vi "ROI group-Update All Groups info.vi"(8 "error in (no error)":errorcluster, 11 "Groups setup to add/update":T1[](array[typedef]) {"Group region specifier cluster"."Contours"."Type" items=["No Selection", "Point", "Line", "Rectangle", "Oval", "Polygon", "Freehand Region", "Annulus", "Unused2", "Unused3", "Broken Line", "Freehand Line", "Rotated Rectangle"]}) -> (0 "error out":errorcluster, 3 "Updated \"All groups\" setup":T1[](array[typedef]) {"Group region specifier cluster"."Contours"."Type" items=["No Selection", "Point", "Line", "Rectangle", "Oval", "Polygon", "Freehand Region", "Annulus", "Unused2", "Unused3", "Broken Line", "Freehand Line", "Rotated Rectangle"]})   [LabVIEW 2013]
uses:
  ROI Selection Interface/ROI group info cluster.ctl
  Typedefs/Get-Set-Clear Control.ctl
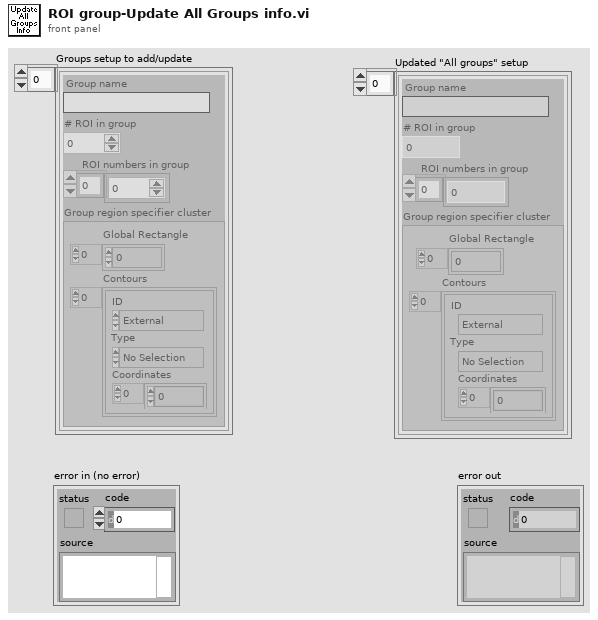
[diagram p1: front panel]
types:
  T1 = typedef "ROI group info cluster.ctl" = cluster{"Group name":string, "# ROI in group":i32, "ROI numbers in group":i32[], "Group region specifier cluster":T2}
  T2 = typedef "ROI Descriptor" = cluster{"Global Rectangle":i32[], "Contours":cluster{"ID":enum32{"External", "Internal"}, "Type":u32, "Coordinates":i32[]}[]}
  T3 = typedef "Get-Set-Clear Control.ctl" = enum16{"Get", "Set", "Clear"}
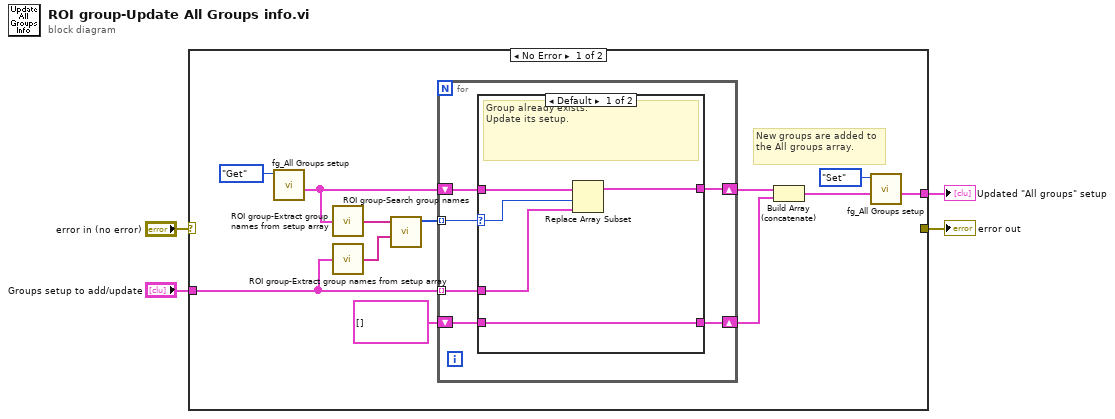
[diagram p0: block diagram]
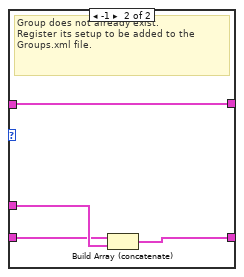
[diagram p2: hidden frame]
diagram:
  n1 = case shown="No Error" "error in (no error)" {
    selector: "error in (no error)" -> [_ w32]
    tunnel: "Groups setup to add/update" -> [w11 _]
    tunnel: [w5 _] -> w3
    tunnel: [_ w32] -> w1
    frame No Error {
      # "New groups are added to the All groups array."
      n2 = call "fg_All Groups setup.vi"("Function"=Get-Set-Clear_Control."Get") -> ("Groups setup out"=w12:T1[])  [unwired: 9 in, 1 out]
      n3 = call "ROI group-Extract group names from setup array.vi"("Groups setup"=w12) -> ("Group Names Array"=w15:string[])
      n4 = call "ROI group-Extract group names from setup array.vi"("Groups setup"=w11) -> ("Group Names Array"=w14:string[])
      n5 = call "ROI group-Search group names.vi"("Group names to search for"=w14, "Group names to search through"=w15) -> ("Indexes (-1 = not found)"=w13:i32[])  [unwired: 9 in]
      n6 = for {
        tunnel: w13 -> [w22] mode=indexing
        tunnel: w11 -> [w20] mode=indexing
        shift-right: [w19] -> w9
        shift-left: w12 -> [w21]
        shift-right: [w18] -> w8
        shift-left: T1[] [] -> [w17]
        n7 = case shown="Default" w22 {
          selector: w22 -> [w26 _]
          tunnel: w21 -> [w27 w31]
          tunnel: w20 -> [w25 w30]
          tunnel: [w24 w31] -> w19
          tunnel: [w23 w29] -> w18
          tunnel: w17 -> [w23 w28]
          frame Default {
            # "Group already exists.\nUpdate its setup."
            n8 = Replace Array Subset(array=w27, new element=w25, index=w26) -> (w24:T1[])
          }
          frame -1 {
            # "Group does not already exist.\nRegister its setup to be added to the Groups.xml file."
            n9 = Build Array (concatenate)(w28, w30) -> (w29:T1[])
          }
        }
      }
      n10 = Build Array (concatenate)(w9, w8) -> (w6:T1[])
      n11 = call "fg_All Groups setup.vi"("Groups setup in"=w6, "Function"=Get-Set-Clear_Control."Set") -> ("Groups setup out"=w5:T1[])  [unwired: 8 in, 1 out]
    }
    frame Error {
    }
  }
  "Updated \"All groups\" setup" <- w3
  "error out" <- w1
